vi "Problem 12.vi"() -> (3 "Triangle Num w/ >500 factors":u64)   [LabVIEW 2013, in "Problem 12.lvlib"]
uses:
  Problem 12.lvlib
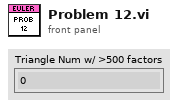
[diagram p1: front panel]
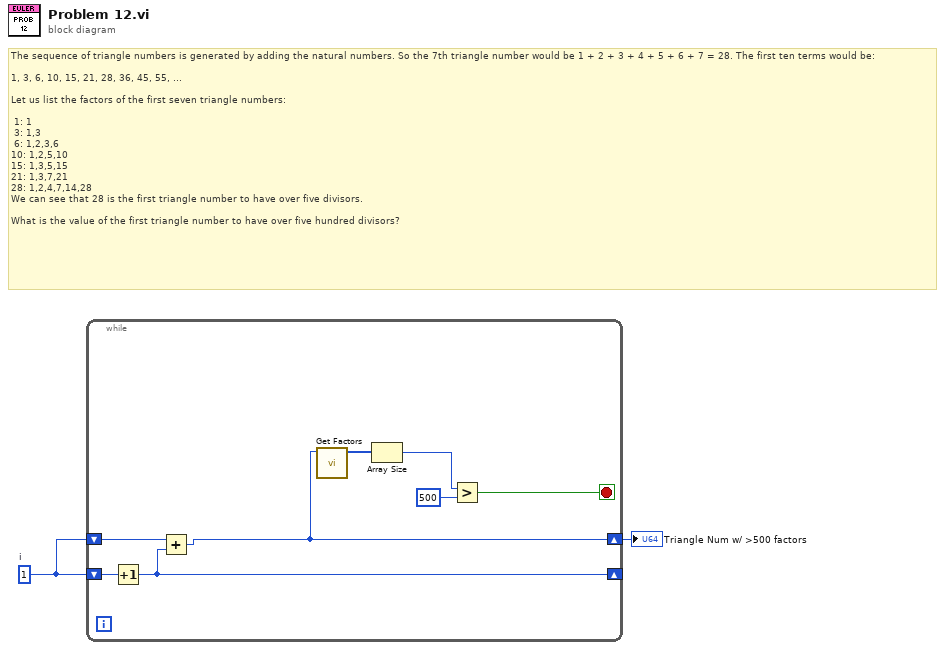
[diagram p0: block diagram]
diagram:
  w2 = u64 1  # i
  # "The sequence of triangle numbers is generated by adding the natural numbers. So the 7th triangle number would be 1 + 2 + 3 + 4 + 5 + 6 + 7 = 28. The first ten terms would be:\n\n1, 3, 6, 10, 15, 21, 28, 36, 45, 55, ...\n\nLet us list the factors of the first seven triangle numbers:\n\n 1: 1\n 3: 1,3\n 6: 1,2,3,6\n10: 1,2,5,10\n15: 1,3,5,15\n21: 1,3,7,21\n28: 1,2,4,7,14,28\nWe can see that 28 is the first triangle number to have over five divisors.\n\nWhat is the value of the first triangle number to have over five hundred divisors?"
  n1 = while {
    shift-right: [w8] -> _
    shift-left: w2 -> [w9]
    shift-right: [w3] -> w1
    shift-left: w2 -> [w10]
    stop <- w6 stop-if-true
    n2 = Increment(x=w9) -> (x+1=w8:u64)
    n3 = Add(x=w10, y=w8) -> (x+y=w3:u64)
    n4 = call "Get Factors.vi"("Number to Factor"=w3) -> ("Factors"=w5:u64[])  [unwired: 10 in]
    n5 = Array Size(array=w5) -> (size(s)=w4:i32)
    n6 = Greater?(x=w4, y=500) -> (0:w6:bool)
  }
  "Triangle Num w/ >500 factors" <- w1
